vi "boarder.vi"(8 "垂直":i32, 11 "水平":i32) -> (0 "垂直out":i32, 3 "水平out":i32)   [LabVIEW 2016]
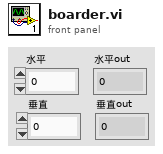
[diagram p1: front panel]
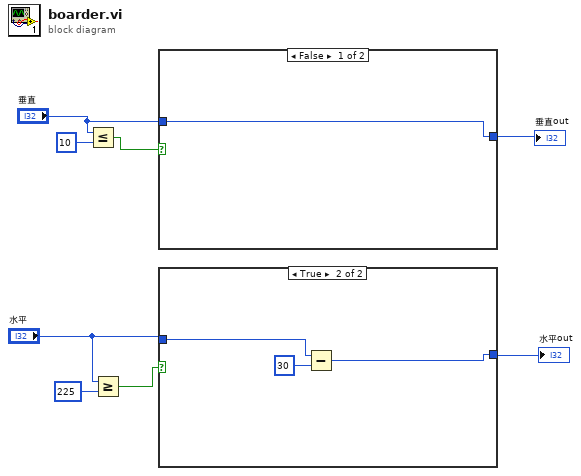
[diagram p0: block diagram]
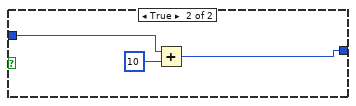
[diagram p3: hidden frame]
diagram:
  n1 = Less Or Equal?(x="垂直", y=10) -> (x <= y?=w7:bool)
  n2 = Greater Or Equal?(x="水平", y=225) -> (x >= y?=w5:bool)
  n3 = case shown="False" w7 {
    tunnel: "垂直" -> [w9 w12]
    tunnel: [w9 w10] -> w3
    frame False {
    }
    frame True {
      n4 = Add(x=w12, y=10) -> (x+y=w10:i32)
    }
  }
  "垂直out" <- w3
  n5 = case shown="True" w5 {
    tunnel: "水平" -> [w13 w16]
    tunnel: [w13 w14] -> w2
    frame False {
    }
    frame True {
      n6 = Subtract(x=w16, y=30) -> (x-y=w14:i32)
    }
  }
  "水平out" <- w2
